vi "Circle0008.vi"   [LabVIEW 2013]
uses:
  <vilib>/Heliosphere Research LLC/Advanced Plotting Toolkit/api_core/NewPlotProperties.ctl
  <vilib>/Heliosphere Research LLC/Advanced Plotting Toolkit/typedefs/PlotColor.ctl
  ModeType.ctl
  <vilib>/Heliosphere Research LLC/Advanced Plotting Toolkit/api_core/NewPlotScales.ctl
  ErrorCodes.ctl
  <vilib>/Heliosphere Research LLC/Advanced Plotting Toolkit/Advanced Plotting Toolkit.lvlib
types:
  T1 = typedef "ErrorCodes.ctl" = u32
  T2 = typedef "Advanced Plotting Toolkit.lvlib/NewPlotScales.ctl" = enum16{"Default", "Linear", "Log", "Symlog"}
  T3 = typedef "ModeType.ctl" = enum16{"Normal", "Expected Failure", "Skipped", "Broken"}
  T4 = typedef "Advanced Plotting Toolkit.lvlib/NewPlotProperties.ctl" = cluster{"Background Color":T5, "Axis Background":T5, "Left Margin":dbl, "Right Margin":dbl, "Bottom Margin":dbl, "Top Margin":dbl, "Aspect Ratio":dbl}
  T5 = typedef "Advanced Plotting Toolkit.lvlib/PlotColor.ctl" = u32
  T6 = typedef "Advanced Plotting Toolkit.lvlib/PlotID.ctl" = i32
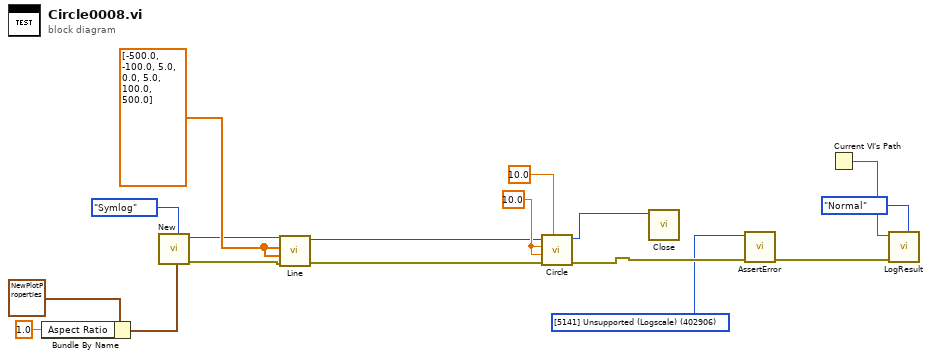
[diagram p0: block diagram]
diagram:
  w1 = T1 402906 items=["[5120] Invalid ID"=402902, "[5110] Failed to Init"=402900, "[5111] Unknown Error"=402901, "[5130] Save - Bad File Extension"=402403, "[5131] Save - General Error"=402904, "[5140] Unsupported (Polar)"=402905, "[5141] Unsupported (Logscale)"=402906, "[5142] Coordinates Not Regular"=402907] ("Expected Error")
  w11 = dbl[] [-500.0, -100.0, 5.0, 0.0, 5.0, 100.0, 500.0] ("X Data")
  w16 = 10.0 ("X Position")
  n1 = Bundle By Name(cluster=T4 {"Background Color"=2147483647, "Axis Background"=2147483647, "Left Margin"=nan, "Right Margin"=nan, "Bottom Margin"=nan, "Top Margin"=nan, "Aspect Ratio"=nan} ("New Plot Properties"), "Aspect Ratio"=1.0) -> (w14:T4)
  n2 = call <vilib>:"New.vi"("Properties"=w14, "Y Axis Scale"=NewPlotScales."Symlog") -> ("error out"=w9:errorcluster, "Plot ID"=w10:T6)  [unwired: 8 in]
  n3 = call <vilib>:"Line.vi"("error in (no error)"=w9, "Y Data"=w11, "X Data"=w11, "Plot ID"=w10) -> ("error out"=w5:errorcluster, "Plot ID out"=w6:T6)  [unwired: 6 in]
  n4 = call <vilib>:"Circle.vi"("Radius"=10.0, "error in (no error)"=w5, "Y Position"=w16, "X Position"=w16, "Plot ID"=w6) -> ("error out"=w4:errorcluster, "Plot ID Out"=w3:T6)  [unwired: 5 in]
  n5 = call <vilib>:"Close.vi"("Plot ID"=w3) -> ()  [unwired: 10 in, 1 out]
  n6 = call "AssertError.vi"("error in (no error)"=w4, "Expected Error"=w1) -> ("error out"=w2:errorcluster)  [unwired: 9 in]
  n7 = Current VI's Path() -> (path=w17:path)
  n8 = call "LogResult.vi"("Mode"=ModeType."Normal", "Test Result"=w2, "VI Path"=w17) -> ()  [unwired: 9 in]
